vi "TIO Data Stream.vi"(1 "Raw Data":T2={"stream ID"=0, "Sample Number"=417475, "Raw Data"=":-É%a\u0000J1\n\u0000É†Eï>tn\u0013Áõ9FÀó\u0010Ÿ<wm\u0010<u;Î;"}, 2 "TIO State":T3={"Awaiting REP"=FALSE, "REQ ID"=500, "streams in"=[], "source"=[], "timebases"=[]}) -> (0 "Data Out":T1(array[cluster])=[{"Name"="gmr", "Waveform"={"start"=0.0, "dt"=1.0, "Timeseries"=[[-1045203.625, 2103369.25, -524451.0625]]}}, {"Name"="accel", "Waveform"={"start"=0.0, "dt"=1.0, "Timeseries"=[[0.4673272967338562, -9.214466094970703, -3.09728741645813]]}}, {"Name"="gyro", "Waveform"={"start"=0.0, "dt"=1.0, "Timeseries"=[[0.019417261704802513, 0.00881516095250845, 0.006293708924204111]]}}, {"Name"="bar", "Waveform"={"start"=0.0, "dt"=1.0, "Timeseries"=[[0.0]]}}, {"Name"="therm", "Waveform"={"start"=0.0, "dt"=1.0, "Timeseries"=[[0.0]]}}])   [LabVIEW 2020]
panel:
  # "TIO Data Stream Process"
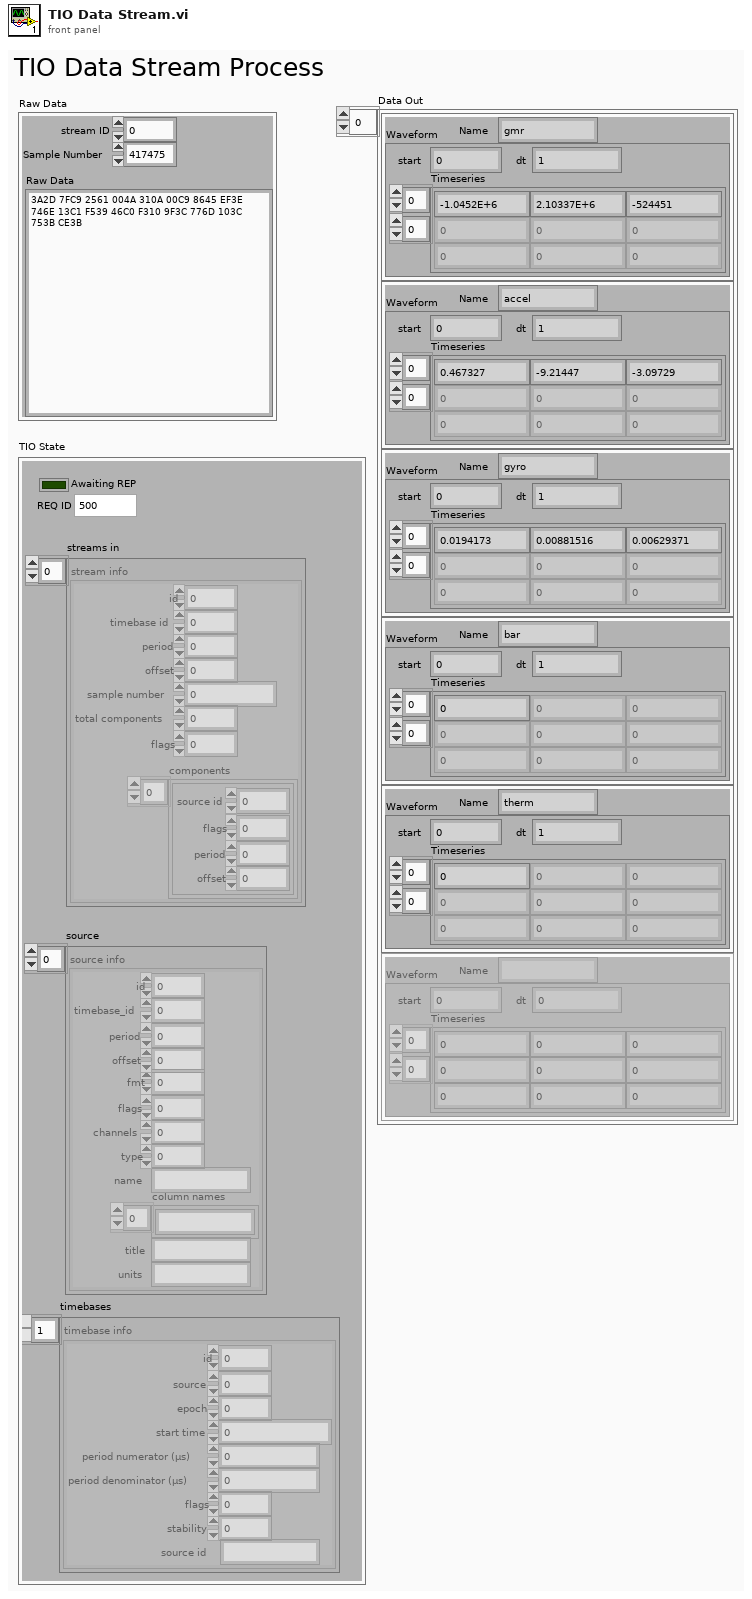
[diagram p1: front panel]
types:
  T1 = cluster{"Name":string, "Waveform":cluster{"start":dbl, "dt":dbl, "Timeseries":dbl[][]}}[]
  T2 = cluster{"stream ID":u16, "Sample Number":u32, "Raw Data":string}
  T3 = cluster{"Awaiting REP":bool, "REQ ID":u32, "streams in":cluster{"id":u16, "timebase id":u16, "period":u32, "offset":u32, "sample number":u64, "total components":u16, "flags":u16, "components":cluster{"source id":u16, "flags":u16, "period":u32, "offset":u32}[]}[], "source":cluster{"id":u16, "timebase_id":u16, "period":u32, "offset":u32, "fmt":i32, "flags":u16, "channels":u16, "type":u8, "name":string, "column names":string[], "title":string, "units":string}[], "timebases":cluster{"id":u16, "source":u8, "epoch":u8, "start time":u64, "period numerator (µs)":u32, "period denominator (µs)":u32, "flags":u32, "stability":sgl, "source id":string}[]}
  T4 = cluster{"id":u16, "source":u8, "epoch":u8, "start time":u64, "period numerator (µs)":u32, "period denominator (µs)":u32, "flags":u32, "stability":sgl, "source id":string}[]
  T5 = cluster{"id":u16, "timebase_id":u16, "period":u32, "offset":u32, "fmt":i32, "flags":u16, "channels":u16, "type":u8, "name":string, "column names":string[], "title":string, "units":string}[]
  T6 = cluster{"id":u16, "timebase id":u16, "period":u32, "offset":u32, "sample number":u64, "total components":u16, "flags":u16, "components":cluster{"source id":u16, "flags":u16, "period":u32, "offset":u32}[]}[]
  T7 = cluster{"id":u16, "timebase id":u16, "period":u32, "offset":u32, "sample number":u64, "total components":u16, "flags":u16, "components":cluster{"source id":u16, "flags":u16, "period":u32, "offset":u32}[]}
  T8 = cluster{"source id":u16, "flags":u16, "period":u32, "offset":u32}[]
  T9 = cluster{"id":u16, "source":u8, "epoch":u8, "start time":u64, "period numerator (µs)":u32, "period denominator (µs)":u32, "flags":u32, "stability":sgl, "source id":string}
  T10 = enum16{"big-endian, network order", "native, host order", "little-endian"}
  T11 = cluster{"id":u16, "timebase_id":u16, "period":u32, "offset":u32, "fmt":i32, "flags":u16, "channels":u16, "type":u8, "name":string, "column names":string[], "title":string, "units":string}
  T12 = cluster{"name":string, cluster{dbl, dbl, dbl[][]}}
  T13 = cluster{"name":string, cluster{dbl, dbl, dbl[][]}}[]
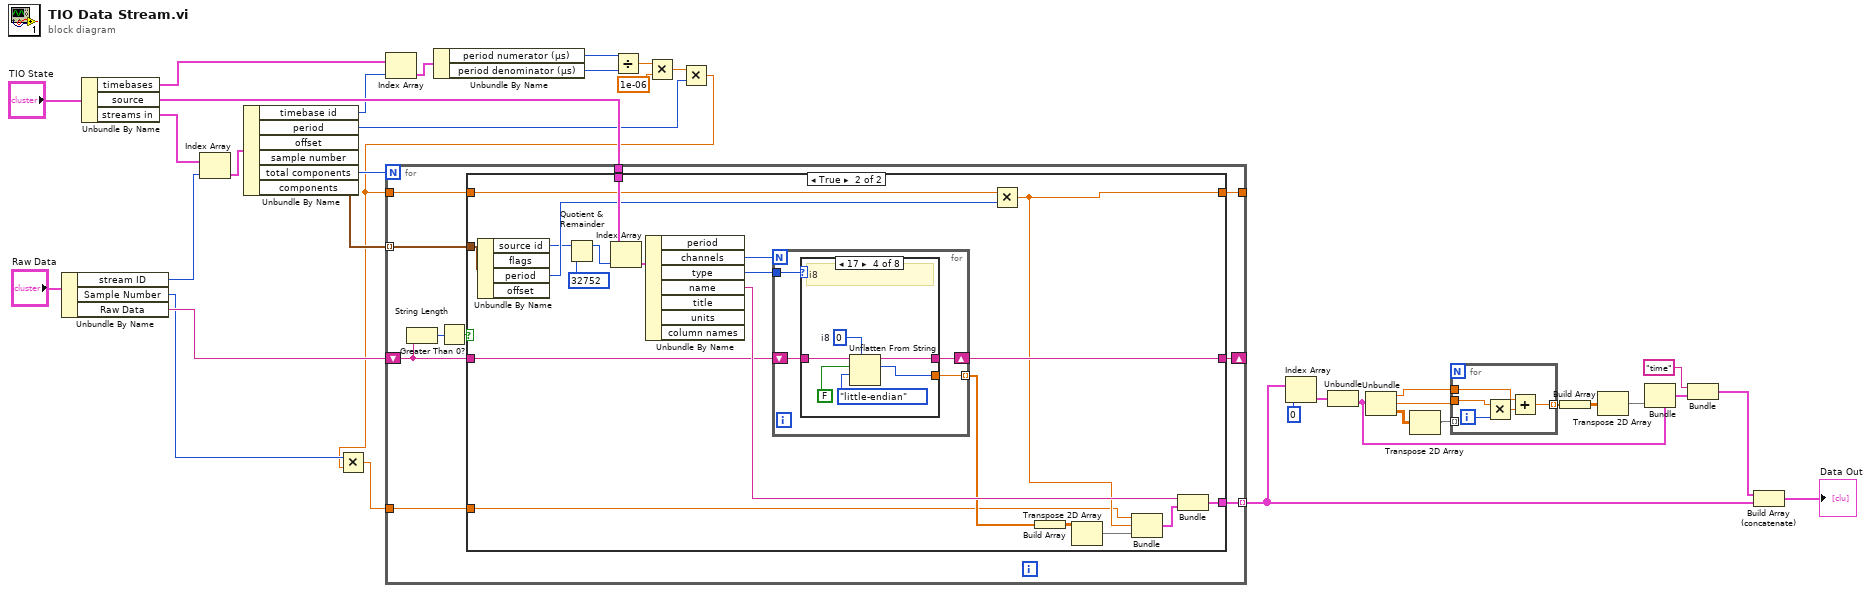
[diagram p0: block diagram]
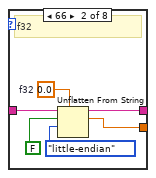
[diagram p4: hidden frame]
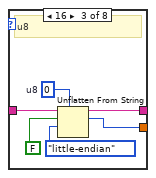
[diagram p5: hidden frame]
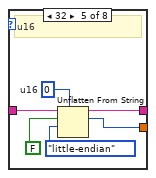
[diagram p6: hidden frame]
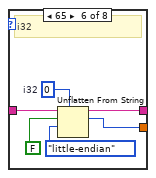
[diagram p7: hidden frame]
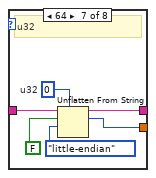
[diagram p8: hidden frame]
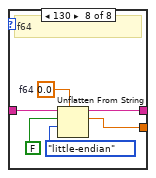
[diagram p9: hidden frame]
diagram:
  n1 = Unbundle By Name("Raw Data") -> ("stream ID"=w34:u16, "Sample Number"=w3:u32, "Raw Data"=w28:string)
  n2 = Unbundle By Name("TIO State") -> ("timebases"=w26:T4, "source"=w29:T5, "streams in"=w33:T6)
  n3 = Index Array(array=w33, index=w34) -> (element=w32:T7)
  n4 = Unbundle By Name(w32) -> ("timebase id"=w27:u16, "period"=w20:u32, "total components"=w31:u16, "components"=w30:T8)  [unwired: 2 out]
  n5 = Index Array(array=w26, index=w27) -> (element=w25:T9)
  n6 = Unbundle By Name(w25) -> ("period numerator (µs)"=w24:u32, "period denominator (µs)"=w23:u32)
  n7 = Divide(x=w24, y=w23) -> (x/y=w22:dbl)
  n8 = Multiply(x=w22, y=1e-06) -> (x*y=w21:dbl)
  n9 = Multiply(x=w21, y=w20) -> (x*y=w1:dbl)
  n10 = Multiply(x=w3, y=w1) -> (x*y=w2:dbl)
  n11 = for {
    N: w31 -> [_]
    tunnel: w30 -> [w46] mode=indexing
    tunnel: w29 -> [w45]
    shift-right: [w44] -> _
    shift-left: w28 -> [w42]
    tunnel: [w43] -> w17 mode=indexing
    tunnel: w2 -> [w37]
    tunnel: w1 -> [w38]
    tunnel: [w39] -> _
    n12 = String Length(string=w42) -> (length=w41:i32)
    n13 = Greater Than 0?(x=w41) -> (x > 0?=w40:bool)
    n14 = case shown="True" w40 {
      tunnel: w46 -> [_ w68]
      tunnel: w45 -> [_ w67]
      tunnel: [w48 w63] -> w44
      tunnel: [_ w61] -> w43
      tunnel: w42 -> [w48 w58]
      tunnel: w38 -> [w47 w55]
      tunnel: [w47 w54] -> w39
      tunnel: w37 -> [_ w53]
      frame False {
      }
      frame True {
        n15 = Unbundle By Name(w68) -> ("source id"=w50:u16, "period"=w52:u32)  [unwired: 2 out]
        n16 = Quotient & Remainder(x=w50, y=u16 32752) -> (x-y*floor(x/y)=w49:u16)  [unwired: 1 out]
        n17 = Index Array(array=w67, index=w49) -> (element=w66:T11)
        n18 = Unbundle By Name(w66) -> ("channels"=w65:u16, "type"=w64:u8, "name"=w62:string)  [unwired: 4 out]
        n19 = for {
          N: w65 -> [_]
          tunnel: w64 -> [w72]
          tunnel: [w71] -> w60 mode=indexing
          shift-right: [w70] -> w63
          shift-left: w58 -> [w69]
          n20 = case shown="17" w72 {
            tunnel: w69 -> [_ w78 w84 w90 w96 w102 w108 w114]
            tunnel: [_ w74 w80 w86 w92 w98 w104 w110] -> w71
            tunnel: [_ w73 w79 w85 w91 w97 w103 w109] -> w70
            frame 0, Default {
            }
            frame 66 {
              w75 = sgl 0.0  # f32
              # "f32"
              n21 = Unflatten From String(type=w75, binary string=w78, data includes array or string size? (T)=FALSE, byte order (0:big-endian, network order)=T10."little-endian") -> (rest of the binary string=w73:string, value=w74:sgl)  [unwired: 1 in, 1 out]
            }
            frame 16 {
              w81 = u8 0  # u8
              # "u8"
              n22 = Unflatten From String(type=w81, binary string=w84, data includes array or string size? (T)=FALSE, byte order (0:big-endian, network order)=T10."little-endian") -> (rest of the binary string=w79:string, value=w80:u8)  [unwired: 1 in, 1 out]
            }
            frame 17 {
              w87 = i8 0  # i8
              # "i8"
              n23 = Unflatten From String(type=w87, binary string=w90, data includes array or string size? (T)=FALSE, byte order (0:big-endian, network order)=T10."little-endian") -> (rest of the binary string=w85:string, value=w86:i8)  [unwired: 1 in, 1 out]
            }
            frame 32 {
              w93 = u16 0  # u16
              # "u16"
              n24 = Unflatten From String(type=w93, binary string=w96, data includes array or string size? (T)=FALSE, byte order (0:big-endian, network order)=T10."little-endian") -> (rest of the binary string=w91:string, value=w92:u16)  [unwired: 1 in, 1 out]
            }
            frame 65 {
              w99 = 0  # i32
              # "i32"
              n25 = Unflatten From String(type=w99, binary string=w102, data includes array or string size? (T)=FALSE, byte order (0:big-endian, network order)=T10."little-endian") -> (rest of the binary string=w97:string, value=w98:i32)  [unwired: 1 in, 1 out]
            }
            frame 64 {
              w105 = u32 0  # u32
              # "u32"
              n26 = Unflatten From String(type=w105, binary string=w108, data includes array or string size? (T)=FALSE, byte order (0:big-endian, network order)=T10."little-endian") -> (rest of the binary string=w103:string, value=w104:u32)  [unwired: 1 in, 1 out]
            }
            frame 130 {
              w111 = 0.0  # f64
              # "f64"
              n27 = Unflatten From String(type=w111, binary string=w114, data includes array or string size? (T)=FALSE, byte order (0:big-endian, network order)=T10."little-endian") -> (rest of the binary string=w109:string, value=w110:dbl)  [unwired: 1 in, 1 out]
            }
          }
        }
        n28 = Multiply(x=w55, y=w52) -> (x*y=w54:dbl)
        n29 = Build Array(w60) -> (w57:dbl[][])
        n30 = Transpose 2D Array(2D array=w57) -> (transposed array=w56:dbl[][])
        n31 = Bundle(w53, w54, w56) -> (w59:cluster{dbl, dbl, dbl[][]})  [unwired: 1 in]
        n32 = Bundle("name"=w62, w59) -> (w61:T12)  [unwired: 1 in]
      }
    }
  }
  n33 = Index Array(array=w17, index=0) -> (element=w15:T12)
  n34 = Unbundle(w15) -> (w12:cluster{dbl, dbl, dbl[][]})  [unwired: 1 out]
  n35 = Unbundle(w12) -> (w13:dbl, w14:dbl, w5:dbl[][])
  n36 = Transpose 2D Array(2D array=w5) -> (transposed array=w4:dbl[][])
  n37 = for {
    tunnel: w13 -> [w116]
    tunnel: w14 -> [w118]
    tunnel: [w115] -> w9 mode=indexing
    tunnel: w4 -> [_] mode=indexing
    i -> [w119]
    n38 = Multiply(x=w118, y=w119) -> (x*y=w117:dbl)
    n39 = Add(x=w116, y=w117) -> (x+y=w115:dbl)
  }
  n40 = Build Array(w9) -> (w8:dbl[][])
  n41 = Transpose 2D Array(2D array=w8) -> (transposed array=w7:dbl[][])
  n42 = Bundle(cluster=w12, w7) -> (w11:cluster{dbl, dbl, dbl[][]})  [unwired: 2 in]
  n43 = Bundle("time", w11) -> (w6:cluster{string, cluster{dbl, dbl, dbl[][]}})  [unwired: 1 in]
  n44 = Build Array (concatenate)(w6, w17) -> (→"Data Out":T13)
